vi "Set Panes to Origin.vi"(8 "Error in":errorcluster caption="Error in (no error)") -> (0 "Error out":errorcluster)   [LabVIEW 2018]
uses:
  <vilib>/Utility/miscctls.llb/LVPointTypeDef.ctl
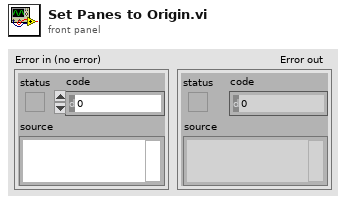
[diagram p1: front panel]
types:
  T1 = typedef "LVPointTypeDef.ctl" = cluster{"Horizontal":i16, "Vertical":i16}
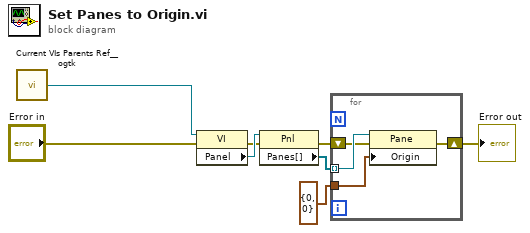
[diagram p0: block diagram]
diagram:
  n1 = call <userlib>:"Current VIs Parents Ref__ogtk.vi"() -> ("Calling VI's Reference"=w5:refnum<vi>)  [unwired: 2 in]
  n2 = property class="VI"(reference=w5, error in="Error in") -> (error out=w3:errorcluster, "Panel"=w6:refnum<vi>)  [unwired: 1 out]
  n3 = property class="Pnl"(reference=w6, error in=w3) -> (error out=w2:errorcluster, "Panes[]"=w7:refnum<vi>[])  [unwired: 1 out]
  n4 = for {
    tunnel: w7 -> [w12] mode=indexing
    tunnel: T1 {"Horizontal"=0, "Vertical"=0} ("Origin") -> [w11]
    shift-right: [w9] -> w1
    shift-left: w2 -> [w10]
    n5 = property class="Pane"(reference=w12, error in=w10, "Origin"=w11) -> (error out=w9:errorcluster)  [unwired: 1 out]
  }
  "Error out" <- w1
